vi "NXT_MIDBRAIN Get Behavior Weights.vi"(2 "_behaviorWeights":T1, 3 "_fromPC":u8[](array[numeric])) -> (0 "_behaviorWeights":T1)   [LabVIEW 2012, in "Tugboat.lvrbt"]
uses:
  Tugboat.lvrbt
  behaviorWeights_t.ctl
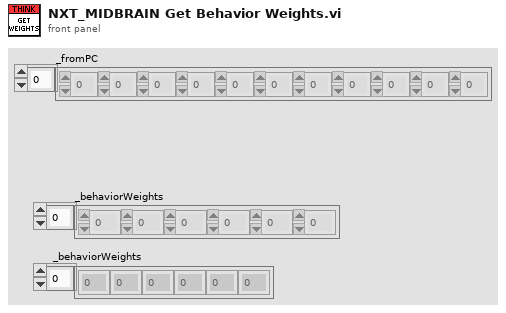
[diagram p1: front panel]
types:
  T1 = typedef "behaviorWeights_t.ctl" = i8[]
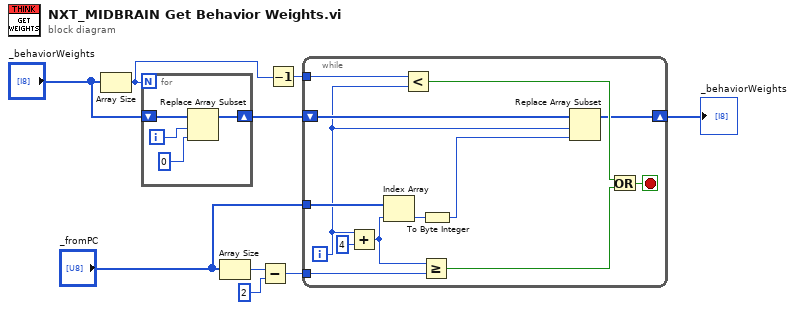
[diagram p0: block diagram]
diagram:
  n1 = Array Size(array="_behaviorWeights") -> (size(s)=w8:i32)
  n2 = for {
    N: w8 -> [_]
    shift-right: [w10] -> w9
    shift-left: "_behaviorWeights" -> [w12]
    i -> [w13]
    n3 = Replace Array Subset(array=w12, new element=0 ("new element/subarray"), index=w13) -> (w10:T1)
  }
  n4 = Array Size(array="_fromPC") -> (size(s)=w4:i32)
  n5 = Subtract(x=w4, y=2 ("x")) -> (x-y=w3:i32)
  n6 = Decrement(x=w8) -> (x-1=w7:i32)
  n7 = while {
    tunnel: w3 -> [w26]
    tunnel: w7 -> [w25]
    shift-right: [w20] -> w5
    shift-left: w9 -> [w21]
    tunnel: "_fromPC" -> [w19]
    i -> [w17]
    stop <- w22 stop-if-true
    n8 = Add(x=w17, y=4) -> (x+y=w15:i32)
    n9 = Index Array(array=w19, index=w15) -> (element=w18:u8)
    n10 = Less?(x=w25, y=w17) -> (x < y?=w23:bool)
    n11 = Greater Or Equal?(x=w15, y=w26) -> (x >= y?=w24:bool)
    n12 = To Byte Integer(number=w18) -> (8bit integer=w14:i8)
    n13 = Replace Array Subset(array=w21, new element=w14, index=w17) -> (w20:T1)
    n14 = Or(x=w23, y=w24) -> (x .or. y?=w22:bool)
  }
  "_behaviorWeights" <- w5
